vi "Build Frequency Array.vi"(1 "f0":dbl, 2 "df":dbl, 3 "pwr spctm length":i32) -> (0 "freq array":dbl[](array[numeric]))   [LabVIEW 2021]
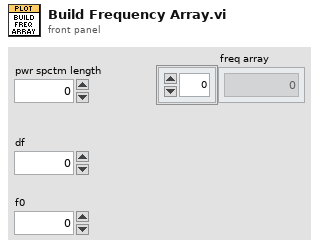
[diagram p1: front panel]
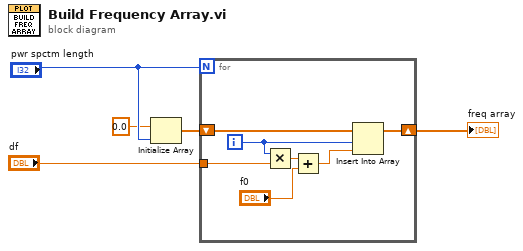
[diagram p0: block diagram]
diagram:
  n1 = Initialize Array(0.0 ("element"), "pwr spctm length") -> (w3:dbl[])
  n2 = for {
    N: "pwr spctm length" -> [_]
    shift-right: [w6] -> w4
    shift-left: w3 -> [w12]
    tunnel: "df" -> [w10]
    i -> [w11]
    n3 = Multiply(x=w11, y=w10) -> (x*y=w9:dbl)
    n4 = Add(x=w9, y="f0") -> (x+y=w7:dbl)
    n5 = Insert Into Array(array=w12, index=w11, new element=w7) -> (w6:dbl[])
  }
  "freq array" <- w4
